vi "Enable High Voltage Channel.vi"(8 "error in (no error)":errorcluster, 10 "Channel (1)":i32=1, 11 "VISA resource name":refnum<visa-resource-name>) -> (0 "error out":errorcluster, 3 "VISA resource name out":refnum<visa-resource-name>)   [LabVIEW 2014, in "Associated Research SC6540.lvlib"]
doc: "Connect the specified channel to high voltage. The other channels will not be changed."
uses:
  <instrlib>/Associated Research SC6540/Associated Research SC6540.lvlib
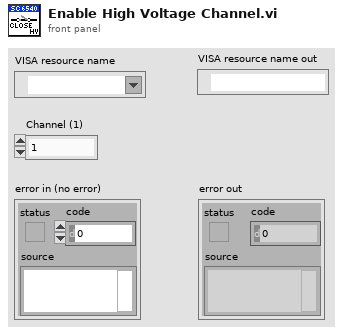
[diagram p1: front panel]
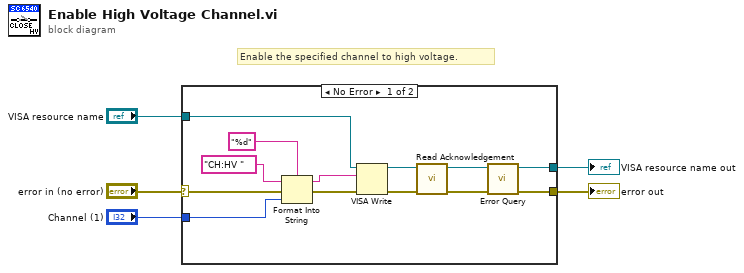
[diagram p0: block diagram]
diagram:
  # "Enable the specified channel to high voltage."
  n1 = case shown="No Error" "error in (no error)" {
    selector: "error in (no error)" -> [w17 w19]
    tunnel: "Channel (1)" -> [w18 _]
    tunnel: "VISA resource name" -> [w13 w20]
    tunnel: [w7 w20] -> w2
    tunnel: [w6 w19] -> w1
    frame No Error {
      n2 = Format Into String(format string="%d", initial string="CH:HV " ("command"), error in=w17, w18) -> (resulting string=w12:string, error out=w16:errorcluster)
      n3 = VISA Write(VISA resource name=w13, write buffer=w12, error in (no error)=w16) -> (VISA resource name out=w11:refnum<visa-resource-name>, error out=w10:errorcluster)  [unwired: 1 out]
      n4 = call <instrlib>:"Read Acknowledgement.vi"("error in (no error)"=w10, "VISA resource name"=w11) -> ("error out"=w8:errorcluster, "VISA resource name out"=w9:refnum<visa-resource-name>)  [unwired: 8 in]
      n5 = call <instrlib>:"Error Query.vi"("error in (no error)"=w8, "VISA resource name"=w9) -> ("error out"=w6:errorcluster, "VISA resource name out"=w7:refnum<visa-resource-name>)  [unwired: 6 in, 2 out]
    }
    frame Error {
    }
  }
  "VISA resource name out" <- w2
  "error out" <- w1
